vi "TCP Server State Machine.vi"(8 "error in":errorcluster, 11 "Vision Server in":refnum<class "Vision Server.lvclass">) -> (0 "error out":errorcluster, 3 "Vision Server out":refnum<class "Vision Server.lvclass">)   [LabVIEW 2016, in "Vision Server.lvclass"]
uses:
  Vision Server.lvclass
  Vision Server.lvclass/Vision Server.ctl
  typedef/Message Type.ctl
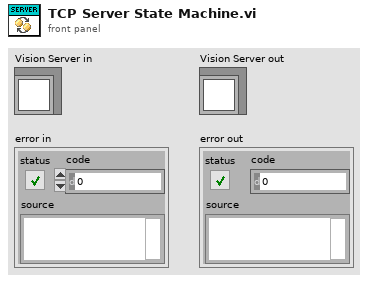
[diagram p1: front panel]
types:
  T1 = enum16{"Standard", "Buffered", "CRLF", "Immediate"}
  T2 = typedef "Vision Server.lvclass/Message Type.ctl" = cluster{"type":string, "message":string}
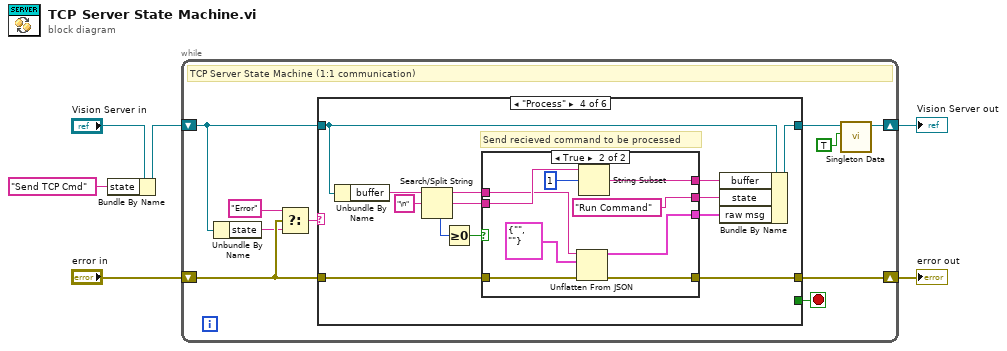
[diagram p0: block diagram]
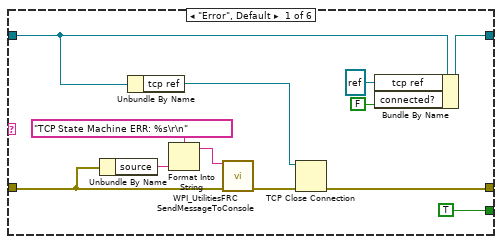
[diagram p2: hidden frame]
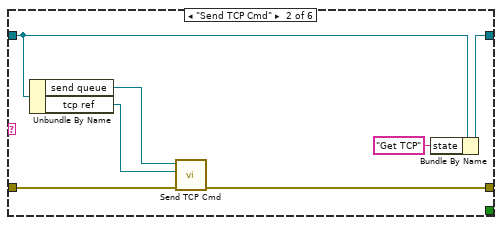
[diagram p3: hidden frame]
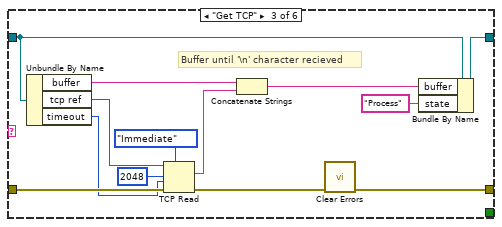
[diagram p4: hidden frame]
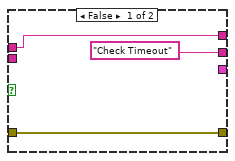
[diagram p5: hidden frame]
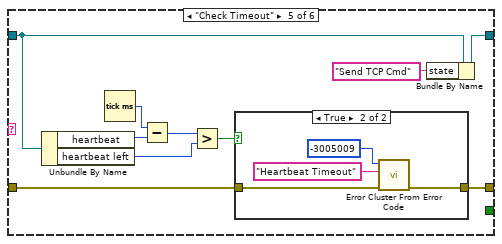
[diagram p6: hidden frame]
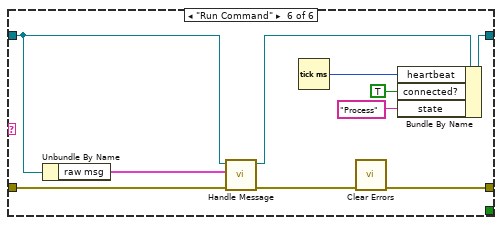
[diagram p8: hidden frame]
diagram:
  n1 = Bundle By Name(cluster="Vision Server in", "state"="Send TCP Cmd") -> (w3:refnum<class "Vision Server.lvclass">)
  n2 = while {
    shift-right: [w16] -> w5
    shift-left: "error in" -> [w13]
    shift-right: [w7] -> w1
    shift-left: w3 -> [w15]
    stop <- w14 stop-if-true
    # "TCP Server State Machine (1:1 communication)"
    n3 = Unbundle By Name(w15) -> ("state"=w12:string)
    n4 = Select(t="Error", s=w13, f=w12) -> (s? t:f=w11:string)
    n5 = case shown="\"Process\"" w11 {
      tunnel: [w24 w30 w37 w56 w80 w91] -> w16
      tunnel: w13 -> [w23 w31 w47 w57 w81 w96]
      tunnel: [w19 w35 w42 w55 w83 w98] -> w8
      tunnel: w15 -> [w21 w33 w43 w59 w79 w93]
      tunnel: [TRUE _ _ _ _ _] -> w14
      frame "Error", Default {
        n6 = Unbundle By Name(w23) -> ("source"=w26:string)
        n7 = Unbundle By Name(w21) -> ("tcp ref"=w20:refnum<k5>)
        n8 = Format Into String(format string="TCP State Machine ERR: %s\r\n", w26) -> (resulting string=w28:string)  [unwired: 2 in, 1 out]
        n9 = call <vilib>:"WPI_UtilitiesFRC SendMessageToConsole.vi"("Message"=w28, "error in (no error)"=w23) -> ("error out"=w25:errorcluster)  [unwired: 13 in]
        n10 = TCP Close Connection(connection ID=w20, error in (no error)=w25) -> (error out=w24:errorcluster)  [unwired: 1 in, 1 out]
        n11 = Bundle By Name(cluster=w21, "tcp ref"=refnum<k5> refnum, "connected?"=FALSE) -> (w19:refnum<class "Vision Server.lvclass">)
      }
      frame "Send TCP Cmd" {
        n12 = Unbundle By Name(w33) -> ("send queue"=w32:refnum<queue>, "tcp ref"=w29:refnum<k5>)
        n13 = call "Send TCP Cmd.vi"("error in"=w31, "tcp ref"=w29, "Queue in"=w32) -> ("error out"=w30:errorcluster)  [unwired: 8 in]
        n14 = Bundle By Name(cluster=w33, "state"="Get TCP") -> (w35:refnum<class "Vision Server.lvclass">)
      }
      frame "Get TCP" {
        # "Buffer until '\\n' character recieved"
        n15 = Unbundle By Name(w43) -> ("buffer"=w40:string, "tcp ref"=w39:refnum<k5>, "timeout"=w38:i32)
        n16 = TCP Read(connection ID=w39, bytes to read=2048, error in (no error)=w47, 7:T1."Immediate" ("mode (standard)"), 9:w38) -> (data out=w44:string, error out=w48:errorcluster)  [unwired: 1 out]
        n17 = Concatenate Strings(w40, w44) -> (w41:string)
        n18 = call <vilib>:"Clear Errors.vi"("error in (no error)"=w48) -> ("error out"=w37:errorcluster)  [unwired: 5 in, 1 out]
        n19 = Bundle By Name(cluster=w43, "buffer"=w41, "state"="Process") -> (w42:refnum<class "Vision Server.lvclass">)
      }
      frame "Process" {
        # "Send recieved command to be processed"
        n20 = Unbundle By Name(w59) -> ("buffer"=w58:string)
        n21 = Search/Split String(string=w58, search string/char (-)="\n") -> (substring before match=w51:string, match + rest of string=w60:string, offset of match=w50:i32)  [unwired: 1 in]
        n22 = Greater Or Equal To 0?(x=w50) -> (x >= 0?=w49:bool)
        n23 = case shown="True" w49 {
          tunnel: w60 -> [_ w73]
          tunnel: w57 -> [w62 w70]
          tunnel: [w62 w69] -> w56
          tunnel: [_ w68] -> w54
          tunnel: ["Check Timeout" ("state") "Run Command" ("state")] -> w53
          tunnel: [w64 w66] -> w52
          tunnel: w51 -> [w64 w65]
          frame False {
          }
          frame True {
            n24 = Unflatten From JSON(JSON string=w65, type and defaults=T2 {"type"="", "message"=""}, error in (no error)=w70) -> (value=w68:T2, error out=w69:errorcluster)  [unwired: 4 in]
            n25 = String Subset(string=w73, offset (0)=1) -> (substring=w66:string)  [unwired: 1 in]
          }
        }
        n26 = Bundle By Name(cluster=w59, "buffer"=w52, "state"=w53, "raw msg"=w54) -> (w55:refnum<class "Vision Server.lvclass">)
      }
      frame "Check Timeout" {
        n27 = Unbundle By Name(w79) -> ("heartbeat"=w77:i32, "heartbeat left"=w75:i32)
        n28 = Tick Count (ms)() -> (millisecond timer value=w78:u32)
        n29 = Subtract(x=w78, y=w77) -> (x-y=w76:u32)
        n30 = Greater?(x=w76, y=w75) -> (0:w74:bool)
        n31 = case shown="True" w74 {
          tunnel: w81 -> [w84 w88]
          tunnel: [w84 w87] -> w80
          frame False {
          }
          frame True {
            n32 = call <vilib>:"Error Cluster From Error Code.vi"("error in (no error)"=w88, "error message (\"\")"="Heartbeat Timeout" ("error message (\"\")"), "error code (0)"=-3005009) -> ("error out"=w87:errorcluster)  [unwired: 6 in]
          }
        }
        n33 = Bundle By Name(cluster=w79, "state"="Send TCP Cmd") -> (w83:refnum<class "Vision Server.lvclass">)
      }
      frame "Run Command" {
        n34 = Unbundle By Name(w93) -> ("raw msg"=w92:T2)
        n35 = call "Handle Message.vi"("error in"=w96, "Message"=w92, "Vision Server in"=w93) -> ("error out"=w95:errorcluster, "Vision Server out"=w90:refnum<class "Vision Server.lvclass">)  [unwired: 7 in]
        n36 = Tick Count (ms)() -> (millisecond timer value=w89:u32)
        n37 = call <vilib>:"Clear Errors.vi"("error in (no error)"=w95) -> ("error out"=w91:errorcluster)  [unwired: 5 in, 1 out]
        n38 = Bundle By Name(cluster=w90, "heartbeat"=w89, "connected?"=TRUE, "state"="Process") -> (w98:refnum<class "Vision Server.lvclass">)
      }
    }
    n39 = call "Singleton Data.vi"("set? (F)"=TRUE, "Vision Server"=w8) -> ("Vision Server Copy"=w7:refnum<class "Vision Server.lvclass">)  [unwired: 8 in, 1 out]
  }
  "Vision Server out" <- w1
  "error out" <- w5
